vi "NodesPropriertysExperiments.vi"() -> ()   [LabVIEW 2018]
panel:
  in  "Slide":dbl(slide) scale=150.0..500.0
  in  "Disabled":T1(ring)
  in  "Visible":bool
  in  "Boolean":bool
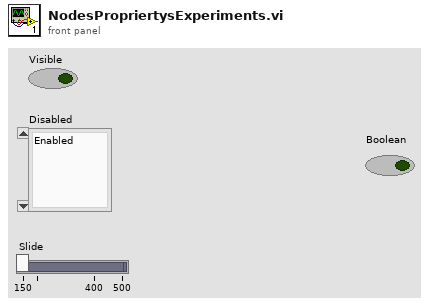
[diagram p1: front panel]
types:
  T1 = enum8{"Enabled", "Disabled", "Disabled and Grayed Out"}
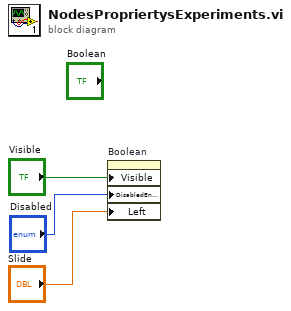
[diagram p0: block diagram]
diagram:
  n1 = property on="Boolean" class="Bool (strict)"("Visible"="Visible", "DisabledEnum"="Disabled", "Left"="Slide") -> ()  [unwired: 2 in, 2 out]
